vi "Set Strings from Ref.vi"(8 "error in (no error)":errorcluster, 9 "Language Index (0)":i32, 10 "GObj Refnum":refnum<vi>, 11 "DiagramText in":refnum<class "StringConstant.lvclass">) -> (0 "error out":errorcluster, 3 "DiagramText out":refnum<class "StringConstant.lvclass">)   [LabVIEW 2013, in "SET Project Data.lvlib" / "StringConstant.lvclass"]
uses:
  StringConstant.lvclass
  GObject/GObject.lvclass
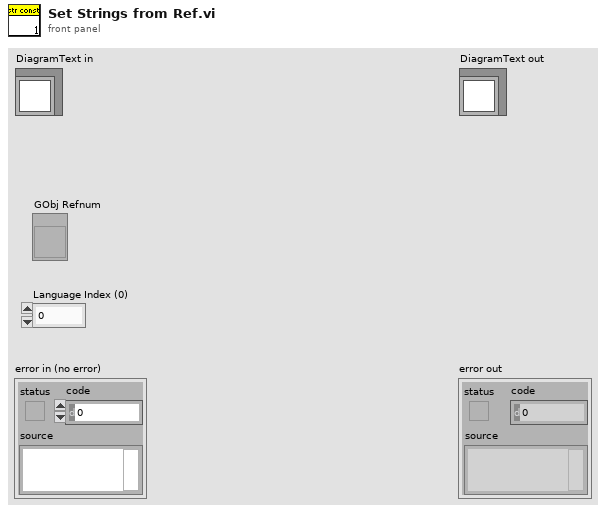
[diagram p1: front panel]
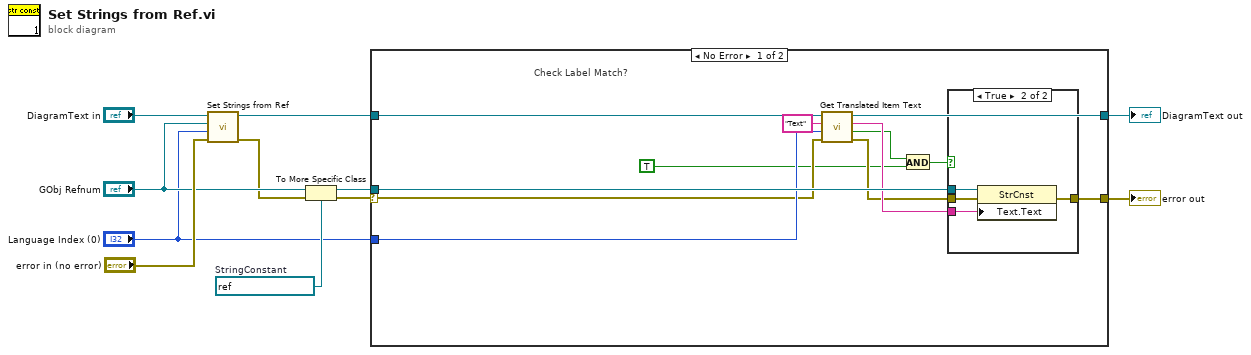
[diagram p0: block diagram]
diagram:
  w5 = refnum<vi> refnum  # StringConstant
  n1 = call-parent "Set Strings from Ref.vi"("error in (no error)"="error in (no error)", "Language Index (0)"="Language Index (0)", "GObj Refnum"="GObj Refnum", "GObject in"="DiagramText in") -> ("error out"=w8:errorcluster, "GObject out"=w4:refnum<class "StringConstant.lvclass">)  [unwired: 6 in]
  n2 = To More Specific Class(target class=w5, reference="GObj Refnum", error in=w8) -> (specific class reference=w6:refnum<vi>, error out=w7:errorcluster)
  n3 = case shown="No Error" w7 {
    selector: w7 -> [w19 w29]
    tunnel: w6 -> [w23 _]
    tunnel: w4 -> [w22 w30]
    tunnel: [w20 w30] -> w3
    tunnel: "Language Index (0)" -> [w21 _]
    tunnel: [w18 w29] -> w1
    frame No Error {
      # "Check Label Match?"
      n4 = call "Get Translated Item Text.vi"("error in (no error)"=w19, "LangIndex (0)"=w21, "ItemName"="Text", "GObject in"=w22) -> ("error out"=w15:errorcluster, "Found?"=w13:bool, "Translated Text (ASCII)"=w16:string, "GObject out"=w20:refnum<class "StringConstant.lvclass">)  [unwired: 4 in]
      n5 = And(x=w13, y=TRUE) -> (x .and. y?=w12:bool)
      n6 = case shown="True" w12 {
        tunnel: w23 -> [_ w28]
        tunnel: w16 -> [_ w27]
        tunnel: w15 -> [w24 w26]
        tunnel: [w24 w25] -> w18
        frame False {
        }
        frame True {
          n7 = property class="StrCnst"(reference=w28, error in=w26, "Text.Text"=w27) -> (error out=w25:errorcluster)  [unwired: 1 out]
        }
      }
    }
    frame Error {
    }
  }
  "error out" <- w1
  "DiagramText out" <- w3
